vi "Write_Data.vi"(8 "error in (no error)":errorcluster caption="entrée d'erreur (pas d'erreur)", 10 "Data_To_Write":string, 11 "Class Instrument Multimeter en entrée":refnum<class "Class Instrument Schielding_Box.lvclass">) -> (0 "error out":errorcluster caption="sortie d'erreur", 3 "Class Instrument Multimeter en sortie":refnum<class "Class Instrument Schielding_Box.lvclass">)   [LabVIEW 2020, in "Library Instrument & Equipement.lvlib" / "Library Instruments.lvlib" / "Class Instrument Schielding_Box.lvclass"]
uses:
  Class Instrument Schielding_Box.lvclass
  Class Instrument Schielding_Box.lvclass/Class Instrument Schielding_Box.ctl
  JSON API/JSON Value/Set from JSON string.vi
  JSON API/JSON Value/JSON Value.lvclass
  JSON API/Variant JSON/Variant JSON.lvlib
  JSON API/Get Polymorphic/JSON GetSet.lvlib
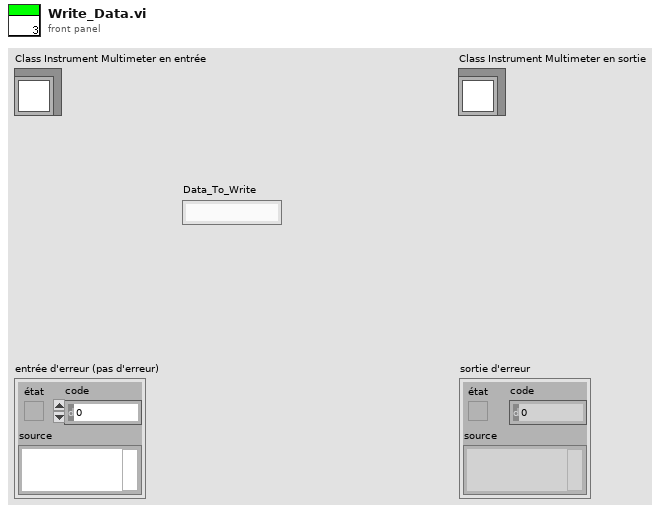
[diagram p1: front panel]
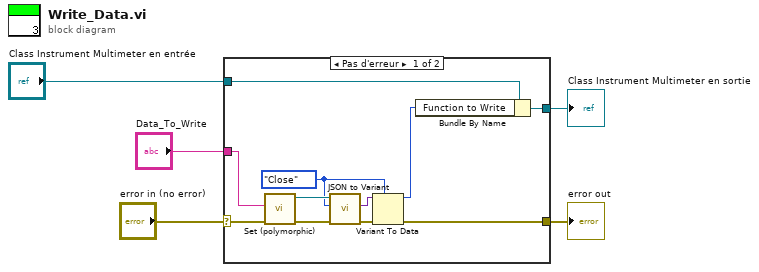
[diagram p0: block diagram]
diagram:
  n1 = case shown="Pas d'erreur" "error in (no error)" {
    selector: "error in (no error)" -> [w11 w18]
    tunnel: [w6 w18] -> w2
    tunnel: [w8 w17] -> w3
    tunnel: "Class Instrument Multimeter en entrée" -> [w9 w17]
    tunnel: "Data_To_Write" -> [w12 _]
    frame No Error {
      w10 = enum16{"Close", "Open"}."Close" ("Status to read")
      n2 = call-poly "Set (polymorphic).vi"("error in (no error)"=w11, "JSON stream"=w12) -> ("error out"=w15:errorcluster, "JSON Value out"=w13:refnum<class "JSON Value.lvclass">)  [unwired: 7 in, 1 out]
      n3 = call "JSON to Variant.vi"("error in (no error)"=w15, "Variant (Data Type)"=w10, "JSON Value"=w13) -> ("error out"=w14:errorcluster, "Variant out"=w16:variant)  [unwired: 7 in]
      n4 = Variant To Data(error in=w14, type=w10, Variant=w16) -> (data=w7:enum16{"Close", "Open"}, error out=w6:errorcluster)
      n5 = Bundle By Name(cluster=w9, "Function to Write"=w7) -> (w8:refnum<class "Class Instrument Schielding_Box.lvclass">)
    }
    frame Error {
    }
  }
  "error out" <- w2
  "Class Instrument Multimeter en sortie" <- w3
